vi "from string 1.0.vi"(8 "error in (no error)":errorcluster, 10 "data":string, 11 "Increment configuration in":refnum<class "Increment configuration.lvclass">) -> (0 "error out":errorcluster, 3 "Increment configuration out":refnum<class "Increment configuration.lvclass">)   [LabVIEW 2015, in "Increment configuration.lvclass"]
uses:
  Increment configuration.lvclass
  <vilib>/NI/Tag Bus Module Framework/channel/TBM channel.lvclass
  Line.ctl
  Increment configuration.lvclass/Increment configuration.ctl
  <vilib>/NI/Configuration Framework/serializable configuration/NISE_CEF_serializable configuration.lvclass
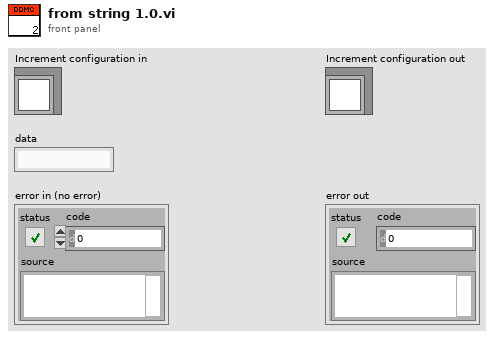
[diagram p1: front panel]
types:
  T1 = typedef "Increment configuration.lvclass/Line.ctl" = cluster{"Name":string, "channel in":refnum<class "TBM channel.lvclass">, "channel out":refnum<class "TBM channel.lvclass">}
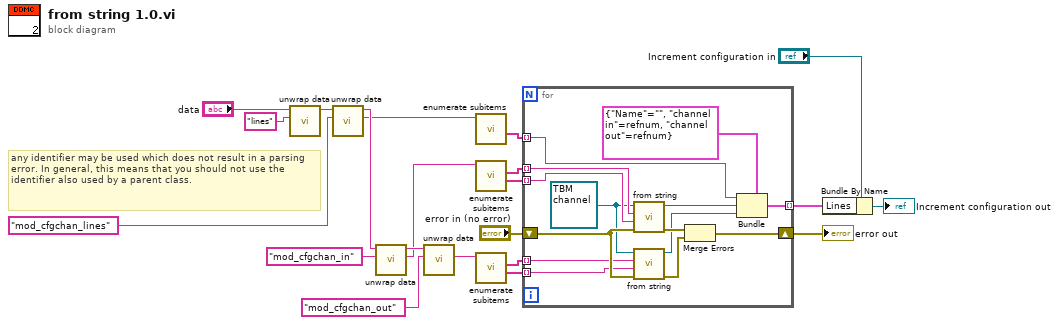
[diagram p0: block diagram]
diagram:
  # "any identifier may be used which does not result in a parsing error. In general, this means that you should not use the identifier also used by a parent class."
  n1 = call <vilib>:"unwrap data.vi"("identifier"="lines" ("additional identifier"), "data to unwrap"="data") -> ("remaining string"=w16:string)  [unwired: 8 in, 1 out]
  n2 = call <vilib>:"unwrap data.vi"("identifier"="mod_cfgchan_lines", "data to unwrap"=w16) -> ("unwrapped data"=w8:string, "remaining string"=w10:string)  [unwired: 8 in]
  n3 = call <vilib>:"unwrap data.vi"("identifier"="mod_cfgchan_in", "data to unwrap"=w10) -> ("unwrapped data"=w7:string, "remaining string"=w9:string)  [unwired: 8 in]
  n4 = call <vilib>:"unwrap data.vi"("identifier"="mod_cfgchan_out", "data to unwrap"=w9) -> ("unwrapped data"=w11:string)  [unwired: 8 in, 1 out]
  n5 = call <vilib>:"enumerate subitems.vi"("data to enumerate"=w8) -> ("associated data"=w6:string[])  [unwired: 8 in, 2 out]
  n6 = call <vilib>:"enumerate subitems.vi"("data to enumerate"=w7) -> ("associated data"=w18:string[], "discovered subitems"=w17:string[])  [unwired: 8 in, 1 out]
  n7 = call <vilib>:"enumerate subitems.vi"("data to enumerate"=w11) -> ("associated data"=w4:string[], "discovered subitems"=w5:string[])  [unwired: 8 in, 1 out]
  n8 = for {
    shift-right: [w27] -> w21
    shift-left: "error in (no error)" -> [w28]
    tunnel: w17 -> [w34] mode=indexing
    tunnel: w18 -> [w33] mode=indexing
    tunnel: [w31] -> w20 mode=indexing
    tunnel: w6 -> [w30] mode=indexing
    tunnel: w5 -> [w25] mode=indexing
    tunnel: w4 -> [w24] mode=indexing
    w22 = refnum<class "TBM channel.lvclass"> refnum ("channel in")
    n9 = call-dynamic "from string.vi"("error in"=w28, "channel data"=w33, "identifier"=w34, "channel in"=w22) -> ("error out"=w35:errorcluster, "channel out"=w29:refnum<class "TBM channel.lvclass">)  [unwired: 6 in]
    n10 = call-dynamic "from string.vi"("error in"=w28, "channel data"=w24, "identifier"=w25, "channel in"=w22) -> ("error out"=w26:errorcluster, "channel out"=w23:refnum<class "TBM channel.lvclass">)  [unwired: 6 in]
    n11 = Merge Errors(w35, w26) -> (w27:errorcluster)
    n12 = Bundle(cluster=T1 {"Name"="", "channel in"=refnum, "channel out"=refnum} ("Line"), "Name"=w30, "channel in"=w29, "channel out"=w23) -> (w31:T1)
  }
  "error out" <- w21
  n13 = Bundle By Name(cluster="Increment configuration in", "Lines"=w20) -> (→"Increment configuration out":refnum<class "Increment configuration.lvclass">)
